vi "myRIO_BRig_Host_formatData_getHeaders_dataAnalog.vi"() -> (3 "output_stringArray_dataAnalog":string[](array[string]))   [LabVIEW 2014]
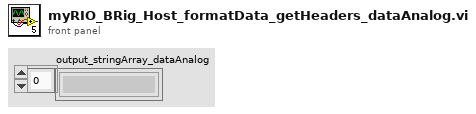
[diagram p1: front panel]
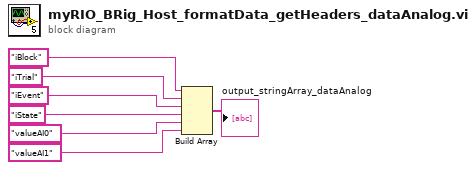
[diagram p0: block diagram]
diagram:
  n1 = Build Array("iBlock", "iTrial", "iEvent", "iState", "valueAI0", "valueAI1") -> (→"output_stringArray_dataAnalog":string[])
